vi "RSNRPZ Zero.vi"(8 "error in (no error)":errorcluster, 10 "Channel (1)":i32=1, 11 "VISA session":refnum<visa-resource-name>) -> (0 "error out":errorcluster, 3 "dup VISA session":refnum<visa-resource-name>)   [LabVIEW 2014]
doc: "This VI performs zeroing of selected sensor using the signal at the sensor input. The sensor must be disconnected from all power sources. If the signal at the input considerably deviates from 0 W, an error message is issued and the command is aborted.\n\nRemote-control command(s):\nSTAT:OPER:MEAS?\nCAL:ZERO:AUTO ONCE"
uses:
  rsnrpz_32.dll
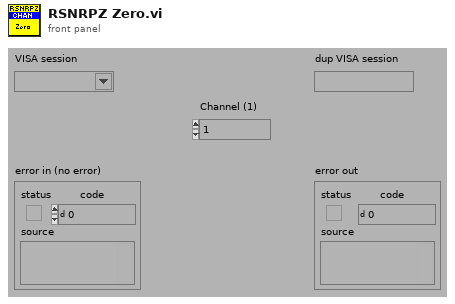
[diagram p1: front panel]
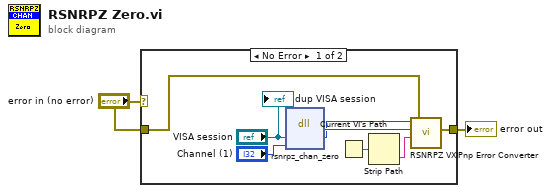
[diagram p0: block diagram]
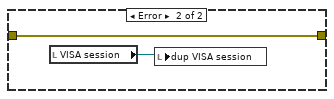
[diagram p2: hidden frame]
diagram:
  n1 = case shown="No Error" "error in (no error)" {
    tunnel: "error in (no error)" -> [w5 w12]
    tunnel: [w6 w12] -> w1
    frame No Error {
      n2 = dll-call lib="rsnrpz_32.dll" fn="rsnrpz_chan_zero"("VISA Session"="VISA session", "Channel"="Channel (1)") -> ("Status"=w9:i32, "VISA Session"=w7:u32)  [unwired: 4 in, 2 out]
      n3 = Current VI's Path() -> (path=w4:path)
      n4 = Strip Path(path=w4) -> (name=w3:string)  [unwired: 1 out]
      n5 = call "RSNRPZ VXIPnp Error Converter.vi"("error in (no error)"=w5, "name of VI"=w3, "VXIPnp error code"=w9, "VISA session"=w7) -> ("error out"=w6:errorcluster)  [unwired: 1 out]
      "dup VISA session" <- "VISA session"
    }
    frame Error {
      n6 = local read "VISA session"() -> (w11:refnum<visa-resource-name>)
      n7 = local write "dup VISA session"(w11) -> ()
    }
  }
  "error out" <- w1
